vi "ADC Read Raw.vi"(8 "error in (no error)":errorcluster, 11 "LINX-ADS1256 in":refnum<class "LINX-ADS1256.lvclass">) -> (0 "error out":errorcluster, 2 "ADC Raw":i32, 3 "LINX-ADS1256 out":refnum<class "LINX-ADS1256.lvclass">)   [LabVIEW 2020, in "LINX-ADS1256.lvclass"]
doc: "Reads the raw ADC value using the RDATA command."
uses:
  LINX-ADS1256.lvclass
  LINX SPI/LINX SPI.lvclass
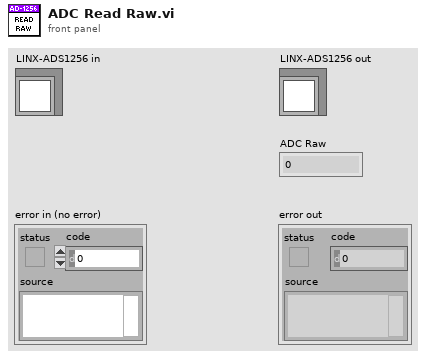
[diagram p1: front panel]
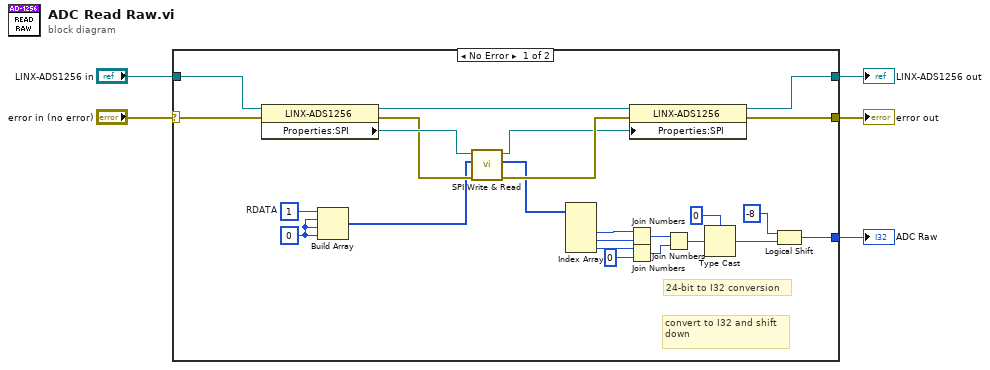
[diagram p0: block diagram]
diagram:
  n1 = case shown="No Error" "error in (no error)" {
    selector: "error in (no error)" -> [w26 w31]
    tunnel: [w25 w31] -> w4
    tunnel: [w27 w30] -> w2
    tunnel: "LINX-ADS1256 in" -> [w29 w30]
    tunnel: [w7 _] -> w1
    frame No Error {
      w19 = u8 0 ("RDATA")
      w20 = u8 1  # RDATA
      # "convert to I32 and shift down"
      # "24-bit to I32 conversion"
      n2 = property class="LINX-ADS1256"(reference=w29, error in=w26) -> (reference out=w28:refnum<class "LINX-ADS1256.lvclass">, error out=w21:errorcluster, "Properties:SPI"=w22:refnum<class "LINX SPI.lvclass">)
      n3 = Build Array(w20, w19, w19, w19) -> (w18:u8[])
      n4 = call "SPI Write & Read.vi"("error in (no error)"=w21, "Data"=w18, "LINX SPI in"=w22) -> ("error out"=w17:errorcluster, "Read Data"=w15:u8[], "LINX SPI out"=w16:refnum<class "LINX SPI.lvclass">)  [unwired: 6 in]
      n5 = Index Array(array=w15) -> (element #2=w12:u8, element #3=w11:u8, element #4=w10:u8)  [unwired: 4 in, 1 out]
      n6 = Join Numbers(hi=w12, lo=w11) -> ((hi.lo)=w14:u16)
      n7 = Join Numbers(hi=w10, lo=u8 0) -> ((hi.lo)=w13:u16)
      n8 = property class="LINX-ADS1256"(reference=w28, error in=w17, "Properties:SPI"=w16) -> (reference out=w27:refnum<class "LINX-ADS1256.lvclass">, error out=w25:errorcluster)
      n9 = Join Numbers(hi=w14, lo=w13) -> ((hi.lo)=w9:u32)
      n10 = Type Cast(type=0 ("ADC Raw"), x=w9) -> (*(type *) &x=w8:i32)
      n11 = Logical Shift(y=-8, x=w8) -> (x << y=w7:i32)
    }
    frame Error {
    }
  }
  "error out" <- w4
  "LINX-ADS1256 out" <- w2
  "ADC Raw" <- w1
